vi "Returning A Value Pointer To Integer.vi"() -> (3 "function return":i32)   [LabVIEW 2018, in "ParsingDataSampleDLL.lvlib"]
doc: "__declspec(dllexport) int* ReturningAValue_PointerToInteger (void);"
uses:
  ParsingDataSampleDLL.lvlib
  ni_reference_vs/Debug/ParsingDataSampleDLL.dll
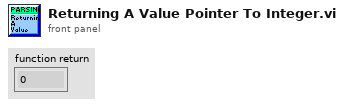
[diagram p1: front panel]
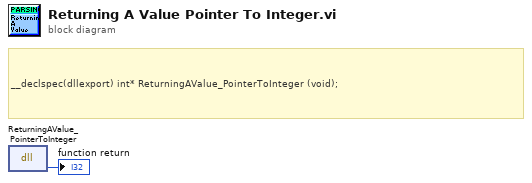
[diagram p0: block diagram]
diagram:
  # "__declspec(dllexport) int* ReturningAValue_PointerToInteger (void);"
  n1 = dll-call lib="C:/Users/celit/Documents/GitHub/Labview_Python_DLL_Call/ni_reference_vs/Debug/ParsingDataSampleDLL.*" fn="ReturningAValue_PointerToInteger"() -> (→"function return":i32)  [unwired: 3 in, 2 out]
